vi "Status Created Events.vi"(11 "Hello World Queue in":refnum<class "Hello World Queue.lvclass">) -> (0 "Created Event Count":i32, 1 "Created Event Aliases":string[](array[string]), 2 "Created Event Exist?":bool, 3 "Hello World Queue out":refnum<class "Hello World Queue.lvclass">)   [LabVIEW 2021, in "Hello World Queue.lvlib" / "Hello World Queue.lvclass"]
uses:
  Hello World Queue.lvclass
  Hello World Queue.lvclass/Hello World Queue.ctl
  jettl/Queue/Queue.lvclass
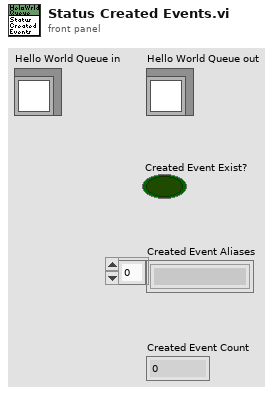
[diagram p1: front panel]
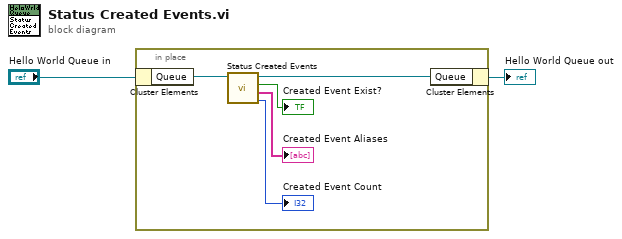
[diagram p0: block diagram]
diagram:
  n1 = in-place {
    n2 = in-place-cluster #1("Hello World Queue in") -> ("Queue"=w7:refnum<class "Queue.lvclass">)
    n3 = call-dynamic "Status Created Events.vi"("Queue in"=w7) -> ("Created Event Count"=→"Created Event Count":i32, "Created Event Aliases"=→"Created Event Aliases":string[], "Created Event Exist?"=→"Created Event Exist?":bool, "Queue out"=w6:refnum<class "Queue.lvclass">)  [unwired: 7 in]
    n4 = in-place-cluster #1("Queue"=w6) -> (→"Hello World Queue out":refnum<class "Hello World Queue.lvclass">)
  }
